vi "ExpEval_EvaluatePostfix.vi"(8 "error in (no error)":errorcluster, 11 "postfix array":string[](array[string])) -> (0 "error out":errorcluster, 3 "result":bool)   [LabVIEW 2017, in "ExpressionEvaluator.lvlib"]
uses:
  <vilib>/addons/InsightCM/Utilities/ExpressionEvaluator/ExpressionEvaluator.lvlib
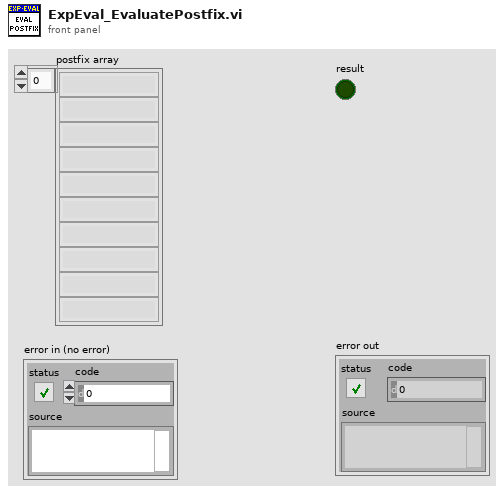
[diagram p1: front panel]
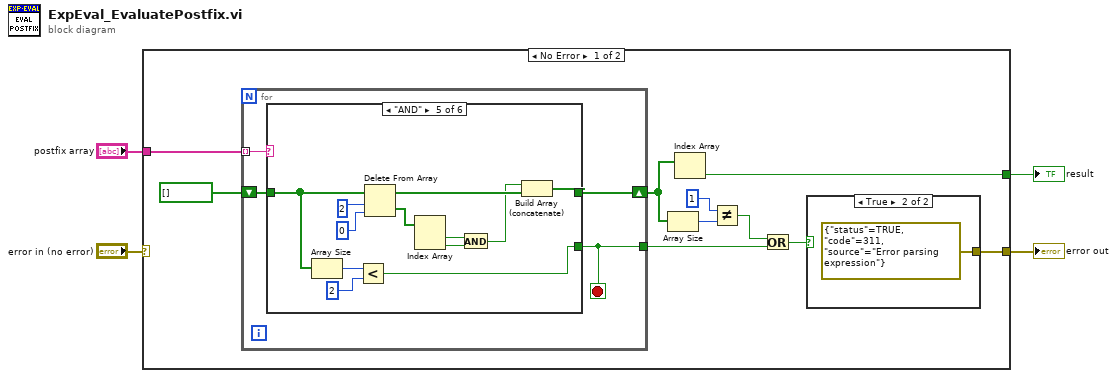
[diagram p0: block diagram]
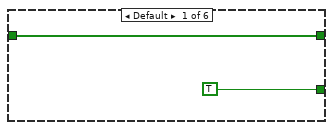
[diagram p3: hidden frame]
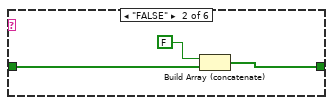
[diagram p4: hidden frame]
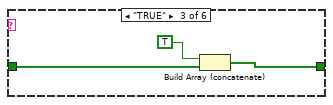
[diagram p5: hidden frame]
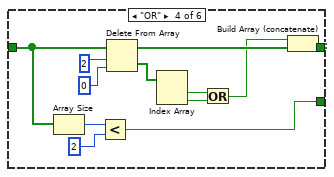
[diagram p6: hidden frame]
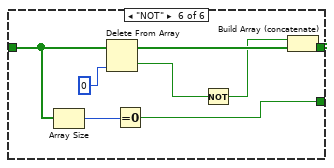
[diagram p7: hidden frame]
diagram:
  n1 = case shown="No Error" "error in (no error)" {
    selector: "error in (no error)" -> [_ w60]
    tunnel: "postfix array" -> [w14 _]
    tunnel: [w12 _] -> w3
    tunnel: [w11 w60] -> w2
    frame No Error {
      n2 = for {
        tunnel: w14 -> [w19] mode=indexing
        shift-right: [w16] -> w10
        shift-left: bool[] [] -> [w17]
        tunnel: [w18] -> w8
        stop <- w18 stop-if-true
        n3 = case shown="\"AND\"" w19 {
          tunnel: [TRUE _ _ w28 w40 w52] -> w18
          tunnel: w17 -> [w20 w24 w27 w29 w43 w54]
          tunnel: [w20 w22 w25 w39 w51 w59] -> w16
          frame Default {
          }
          frame "FALSE" {
            n4 = Build Array (concatenate)(FALSE, w24) -> (w22:bool[])
          }
          frame "TRUE" {
            n5 = Build Array (concatenate)(TRUE, w27) -> (w25:bool[])
          }
          frame "OR" {
            n6 = Array Size(array=w29) -> (size(s)=w31:i32)
            n7 = Less?(x=w31, y=2) -> (x < y?=w28:bool)
            n8 = Delete From Array(array=w29, length=2, index=0) -> (deleted portion=w35:bool[], array with subset deleted=w36:bool[])
            n9 = Index Array(array=w35) -> (element #1=w34:bool, element #2=w33:bool)  [unwired: 2 in]
            n10 = Or(x=w34, y=w33) -> (x .or. y?=w32:bool)
            n11 = Build Array (concatenate)(w32, w36) -> (w39:bool[])
          }
          frame "AND" {
            n12 = Array Size(array=w43) -> (size(s)=w42:i32)
            n13 = Less?(x=w42, y=2) -> (x < y?=w40:bool)
            n14 = Delete From Array(array=w43, length=2, index=0) -> (deleted portion=w47:bool[], array with subset deleted=w48:bool[])
            n15 = Index Array(array=w47) -> (element #1=w46:bool, element #2=w45:bool)  [unwired: 2 in]
            n16 = And(x=w46, y=w45) -> (x .and. y?=w44:bool)
            n17 = Build Array (concatenate)(w44, w48) -> (w51:bool[])
          }
          frame "NOT" {
            n18 = Array Size(array=w54) -> (size(s)=w53:i32)
            n19 = Delete From Array(array=w54, index=0) -> (deleted portion=w55:bool, array with subset deleted=w57:bool[])  [unwired: 1 in]
            n20 = Equal To 0?(x=w53) -> (x = 0?=w52:bool)
            n21 = Not(x=w55) -> (.not. x?=w56:bool)
            n22 = Build Array (concatenate)(w56, w57) -> (w59:bool[])
          }
        }
      }
      n23 = Array Size(array=w10) -> (size(s)=w7:i32)
      n24 = Index Array(array=w10) -> (element=w12:bool)  [unwired: 1 in]
      n25 = Not Equal?(x=1, y=w7) -> (x != y?=w5:bool)
      n26 = Or(x=w5, y=w8) -> (x .or. y?=w9:bool)
      n27 = case shown="True" w9 {
        tunnel: [_ errorcluster {"status"=TRUE, "code"=311, "source"="Error parsing expression"} ("error constant")] -> w11
        frame False {
        }
        frame True {
        }
      }
    }
    frame Error {
    }
  }
  "result" <- w3
  "error out" <- w2
